vi "WLAN ModAcc Configure.vi"(0 "Instrument Handle In":refnum<k21>, 1 "Selector String":string, 5 "ModAcc Configuration":T1={"Acquisition Length (s)"=0.0, "Measurement Config"={"Measurement Offset (symbols)"=0, "Maximum Measurement Length (symbols)"=16}, "Optimize Dynamic Range Config"={"Optimize Dynamic Range for EVM Enabled"=0, "Optimize Dynamic Range for EVM Margin (dB)"=0.0}, "Averaging Config"={"Averaging Enabled"=0, "Averaging Count"=10}} {"Acquisition Length (s)" format="%.3p"; "Averaging Config"."Averaging Enabled" items=["False", "True"]; "Optimize Dynamic Range Config"."Optimize Dynamic Range for EVM Margin (dB)" format="%.2f"; "Optimize Dynamic Range Config"."Optimize Dynamic Range for EVM Enabled" items=["False", "True"]}, 11 "error in (no error)":errorcluster) -> (4 "Instrument Handle Out":refnum<k21>, 15 "error out":errorcluster)   [LabVIEW 2018, in "RFmxWLAN.lvlib"]
uses:
  RFmxWLAN.lvlib
  Typedefs/WLAN ModAcc Config.ctl
  <resource>/objmgr/RFmxWLAN.rc
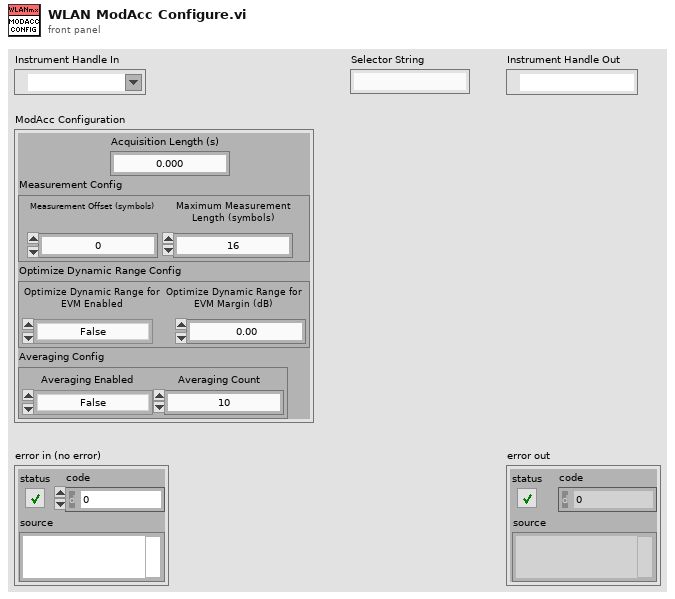
[diagram p1: front panel]
types:
  T1 = typedef "RFmxWLAN.lvlib/WLAN ModAcc Config.ctl" = cluster{"Acquisition Length (s)":dbl, "Measurement Config":cluster{"Measurement Offset (symbols)":i32, "Maximum Measurement Length (symbols)":i32}, "Optimize Dynamic Range Config":cluster{"Optimize Dynamic Range for EVM Enabled":i32, "Optimize Dynamic Range for EVM Margin (dB)":dbl}, "Averaging Config":cluster{"Averaging Enabled":i32, "Averaging Count":i32}}
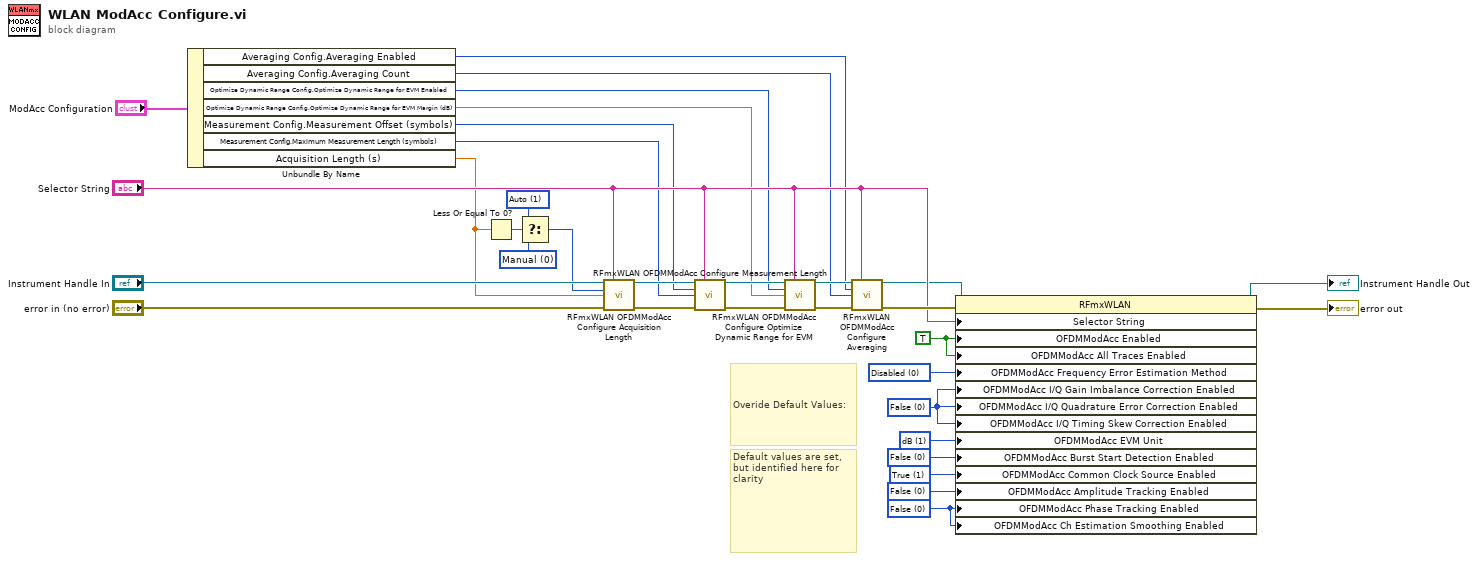
[diagram p0: block diagram]
diagram:
  w12 = 1 items=["Manual", "Auto"] ("Acquisition Length Mode")
  w10 = 0 items=["Manual", "Auto"] ("Acquisition Length Mode")
  w27 = 0 items=["False", "True"] ("OFDMModAcc Amplitude Tracking Enabled")
  w28 = 0 items=["False", "True"] ("OFDMModAcc Amplitude Tracking Enabled")
  w29 = 1 items=["False", "True"] ("OFDMModAcc Burst Start Detection Enabled")
  w30 = 0 items=["False", "True"] ("OFDMModAcc Burst Start Detection Enabled")
  w31 = 1 items=["Percentage", "dB"] ("OFDMModAcc EVM Unit")
  w32 = 0 items=["False", "True"] ("OFDMModAcc I/Q Quadrature Error Correction Enabled")
  w33 = 0 items=["Disabled", "Initial Preamble", "Preamble", "Preamble and Pilots", "Preamble, Pilots and Data"] ("OFDMModAcc Frequency Error Estimation Method")
  w24 = TRUE ("OFDMModAcc Enabled")
  # "Default values are set, but identified here for clarity"
  # "Overide Default Values:"
  n1 = Unbundle By Name("ModAcc Configuration") -> ("Averaging Config.Averaging Enabled"=w3:i32, "Averaging Config.Averaging Count"=w4:i32, "Optimize Dynamic Range Config.Optimize Dynamic Range for EVM Enabled"=w5:i32, "Optimize Dynamic Range Config.Optimize Dynamic Range for EVM Margin (dB)"=w6:dbl, "Measurement Config.Measurement Offset (symbols)"=w8:i32, "Measurement Config.Maximum Measurement Length (symbols)"=w7:i32, "Acquisition Length (s)"=w1:dbl)
  n2 = Less Or Equal To 0?(x=w1) -> (x <= 0?=w13:bool)
  n3 = Select(t=w12, s=w13, f=w10) -> (s? t:f=w11:i32)
  n4 = call <vilib>:"RFmxWLAN OFDMModAcc Configure Acquisition Length.vi"("Instrument Handle In"="Instrument Handle In", "Selector String"="Selector String", "Acquisition Length Mode"=w11, "Acquisition Length (s)"=w1, "error in (no error)"="error in (no error)") -> ("Instrument Handle Out"=w20:refnum<k21>, "error out"=w19:errorcluster)  [unwired: 9 in]
  n5 = call <vilib>:"RFmxWLAN OFDMModAcc Configure Measurement Length.vi"("Instrument Handle In"=w20, "Selector String"="Selector String", "Measurement Offset (symbols)"=w8, "Maximum Measurement Length (symbols)"=w7, "error in (no error)"=w19) -> ("Instrument Handle Out"=w22:refnum<k21>, "error out"=w21:errorcluster)  [unwired: 9 in]
  n6 = call <vilib>:"RFmxWLAN OFDMModAcc Configure Optimize Dynamic Range for EVM.vi"("Instrument Handle In"=w22, "Selector String"="Selector String", "Optimize Dynamic Range for EVM Enabled"=w5, "Optimize Dynamic Range for EVM Margin (dB)"=w6, "error in (no error)"=w21) -> ("Instrument Handle Out"=w18:refnum<k21>, "error out"=w17:errorcluster)  [unwired: 9 in]
  n7 = call <vilib>:"RFmxWLAN OFDMModAcc Configure Averaging.vi"("Instrument Handle In"=w18, "Selector String"="Selector String", "Averaging Enabled"=w3, "Averaging Count"=w4, "error in (no error)"=w17) -> ("Instrument Handle Out"=w2:refnum<k21>, "error out"=w23:errorcluster)  [unwired: 9 in]
  n8 = property class="RFmxWLAN"(reference=w2, error in=w23, "Selector String"="Selector String", "OFDMModAcc Enabled"=w24, "OFDMModAcc All Traces Enabled"=w24, "OFDMModAcc Frequency Error Estimation Method"=w33, "OFDMModAcc I/Q Gain Imbalance Correction Enabled"=w32, "OFDMModAcc I/Q Quadrature Error Correction Enabled"=w32, "OFDMModAcc I/Q Timing Skew Correction Enabled"=w32, "OFDMModAcc EVM Unit"=w31, "OFDMModAcc Burst Start Detection Enabled"=w30, "OFDMModAcc Common Clock Source Enabled"=w29, "OFDMModAcc Amplitude Tracking Enabled"=w28, "OFDMModAcc Phase Tracking Enabled"=w27, "OFDMModAcc Ch Estimation Smoothing Enabled"=w27) -> (reference out=→"Instrument Handle Out":refnum<k21>, error out=→"error out":errorcluster)
